vi "setName.vi"(8 "error in (no error)":errorcluster, 10 "Name in":string, 11 "IComponent in":refnum<class "IComponent.lvclass">) -> (0 "error out":errorcluster, 3 "IComponent out":refnum<class "IComponent.lvclass">)   [LabVIEW 2022 SP3, in "openDAQ.lvlib" / "IBaseObject.lvlib" / "IPropertyObject.lvlib" / "IComponent.lvlib" / "IComponent.lvclass"]
uses:
  <instrlib>/openDAQ/Public/Classes/IComponent/IComponent.lvclass
  <instrlib>/openDAQ/Public/Classes/IComponent/IComponent.lvclass/IComponent.ctl
  <instrlib>/openDAQ/Public/Classes/daqCoreTypes/IString/IString.lvclass
  <instrlib>/openDAQ/Binaries/Windows/x86/copendaq32.dll
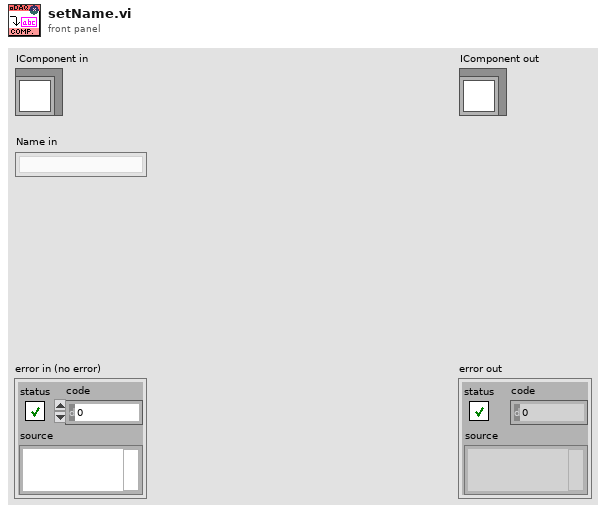
[diagram p1: front panel]
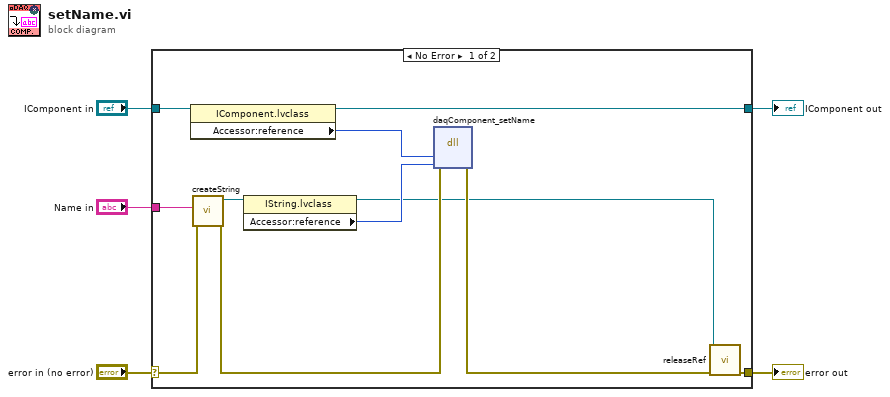
[diagram p0: block diagram]
diagram:
  n1 = case shown="No Error" "error in (no error)" {
    selector: "error in (no error)" -> [w8 w18]
    tunnel: [w9 w18] -> w4
    tunnel: [w13 w17] -> w2
    tunnel: "IComponent in" -> [w14 w17]
    tunnel: "Name in" -> [w11 _]
    frame No Error {
      n2 = property class="IComponent.lvclass"(reference=w14) -> (reference out=w13:refnum<class "IComponent.lvclass">, "Accessor:reference"=w10:i64)  [unwired: 1 in, 1 out]
      n3 = call <instrlib>:"createString.vi"("error in (no error)"=w8, "String"=w11) -> ("error out"=w16:errorcluster, "IString out"=w12:refnum<class "IString.lvclass">)  [unwired: 8 in]
      n4 = property class="IString.lvclass"(reference=w12) -> (reference out=w6:refnum<class "IString.lvclass">, "Accessor:reference"=w15:i64)  [unwired: 1 in, 1 out]
      n5 = dll-call lib="C:/Program Files (x86)/National Instruments/LabVIEW 2022/instr.lib/openDAQ/Binaries/Windows/x86/copendaq*.*" fn="daqComponent_setName"(error in=w16, "component"=w10, "name"=w15) -> (error out=w7:errorcluster)  [unwired: 5 in, 1 out]
      n6 = call-dynamic "releaseRef.vi"("error in (no error)"=w7, "IBaseObject in"=w6) -> ("error out"=w9:errorcluster)  [unwired: 9 in]
    }
    frame Error {
    }
  }
  "error out" <- w4
  "IComponent out" <- w2
